vi "Read inputs.vi"(8 "error in":errorcluster, 11 "shared memory module runtime":refnum<class "Shared Memory Runtime.lvclass">) -> (0 "error out":errorcluster, 2 "inputs":T1[](array[typedef]), 3 "shared memory module runtime out":refnum<class "Shared Memory Runtime.lvclass">)   [LabVIEW 2013, in "Shared Memory Runtime.lvclass"]
doc: "Copyright 2016 National Instruments Corporation\n\nLicensed under the Apache License, Version 2.0 (the \"License\"); you may not use this file except in compliance with the License. You may obtain a copy of the License at http://www.apache.org/licenses/LICENSE-2.0\nUnless required by applicable law or agreed to in writing, software distributed under the License is distributed on an \"AS IS\" BASIS, WITHOUT WARRANTIES OR CONDITIONS OF ANY KIND, either express or implied. See the License for the specific language governing permissions and limitations under the License."
uses:
  Shared Memory Runtime.lvclass
  shared memory module runtime.ctl
  <vilib>/NI/Tag Bus/tag/Data Type.ctl
  Shared Memory Runtime.lvclass/Shared Memory Runtime.ctl
  <vilib>/NI/Tag Bus/tag/tag descriptor.lvclass
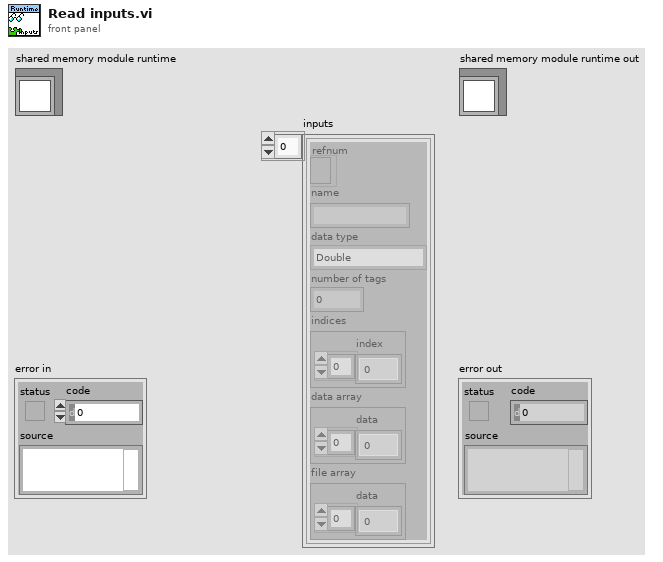
[diagram p1: front panel]
types:
  T1 = typedef "Shared Memory Runtime.lvclass/shared memory module runtime.ctl" = cluster{"refnum":refnum<file>, "name":string, "data type":T2, "number of tags":i32, "indices":cluster{"index":i32[]}, "data array":cluster{"data":dbl[]}, "file array":cluster{"data":dbl[]}}
  T2 = typedef "tag bus.lvlib/tag descriptor.lvclass/Data Type.ctl" = enum16{"Double", "Single", "I64", "I32", "I16", "I8", "U64", "U32", "U16", "U8", "Boolean", "String", "Array of Double", "Array of Single", "Array of I64", "Array of I32", "Array of I16", "Array of I8", "Array of U64", "Array of U32", "Array of U16", "Array of U8", "Array of Boolean", "Array of String"}
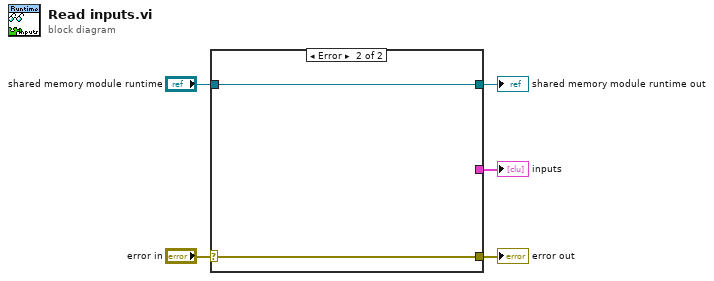
[diagram p0: block diagram]
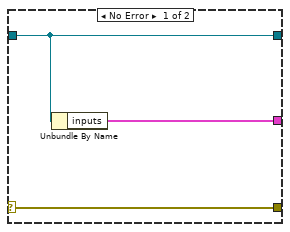
[diagram p2: hidden frame]
diagram:
  n1 = case shown="Error" "error in" {
    selector: "error in" -> [w8 w9]
    tunnel: [w8 w9] -> w4
    tunnel: [w7 w10] -> w2
    tunnel: "shared memory module runtime" -> [w7 w10]
    tunnel: [w6 _] -> w1
    frame No Error {
      n2 = Unbundle By Name(w7) -> ("inputs"=w6:T1[])
    }
    frame Error {
    }
  }
  "error out" <- w4
  "shared memory module runtime out" <- w2
  "inputs" <- w1
